vi "Find All Device of Type X.vi"(0 "Unique Notifier Names":string[](array[string]), 11 "Device Type":T1=enum."Stage") -> (8 "Running Devices":string[](array[string]), 13 "All Devices":string[](array[string]))   [LabVIEW 2016]
uses:
  Hardware Configuration Controls/Device Type.ctl
  <vilib>/regexp/Match Regular Expression.xnode
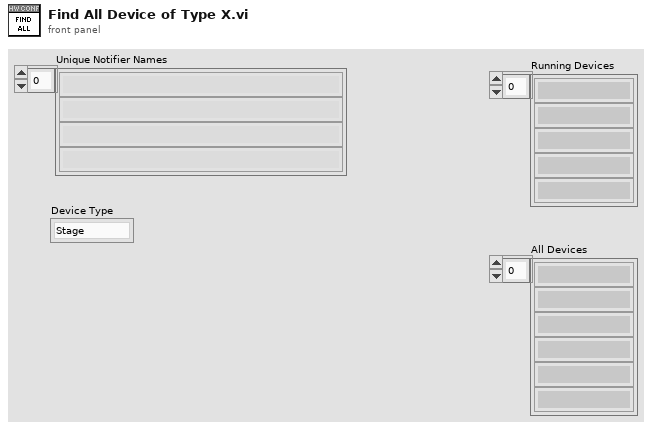
[diagram p1: front panel]
types:
  T1 = typedef "Device Type.ctl" = enum16{"AOTF", "Camera", "Deformable Mirror", "Laser", "Shutter", "Stage", "Waveform", "FPGA", "Email", "Filter Wheel"}
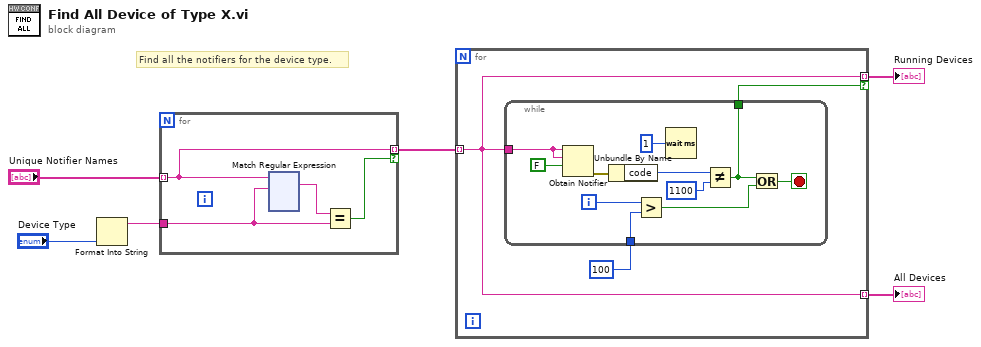
[diagram p0: block diagram]
diagram:
  # "Find all the notifiers for the device type."
  n1 = Format Into String("Device Type") -> (resulting string=w4:string)  [unwired: 3 in, 1 out]
  n2 = for {
    tunnel: "Unique Notifier Names" -> [w9] mode=indexing
    tunnel: [w9] -> w3 mode=indexing if=w8
    tunnel: w4 -> [w7]
    n3 = xnode "Match Regular Expression"("input string"=w9, "regular expression"=w7) -> ("whole match"=w10:string)  [unwired: 4 in, 4 out]
    n4 = Equal?(x=w10, y=w7) -> (x = y?=w8:bool)
  }
  n5 = for {
    tunnel: w3 -> [w125] mode=indexing
    tunnel: [w125] -> w2 mode=indexing if=w126
    tunnel: [w125] -> w1 mode=indexing
    n6 = while {
      tunnel: [w130] -> w126
      tunnel: 100 ("Wait Time (ms)") -> [w129]
      tunnel: w125 -> [w128]
      i -> [w136]
      stop <- w131 stop-if-true
      n7 = Obtain Notifier(name (unnamed)=w128, notification data type=w128, create if not found? (T)=FALSE) -> (error out=w137:errorcluster)  [unwired: 1 in, 2 out]
      n8 = Unbundle By Name(w137) -> ("code"=w135:i32)
      n9 = Greater?(x=w136, y=w129) -> (0:w132:bool)
      n10 = Wait (ms)(milliseconds to wait=u32 1) -> ()  [unwired: 1 out]
      n11 = Not Equal?(x=w135, y=1100) -> (x != y?=w130:bool)
      n12 = Or(x=w130, y=w132) -> (x .or. y?=w131:bool)
    }
  }
  "Running Devices" <- w2
  "All Devices" <- w1
